vi "Phase unwrap (degrees).vi"(1 "Phase Shift (phy)\n(degrees)":dbl format="%#_6f") -> (0 "Degree":dbl)   [LabVIEW 2009]
panel:
  out "Principal value of\nphase shift":dbl
  out "(radians)":dbl
  # "radian"
  # "="
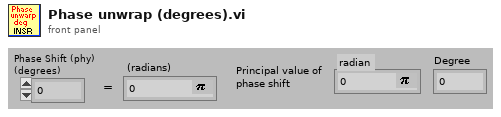
[diagram p1: front panel]
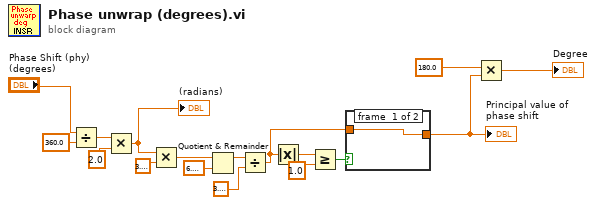
[diagram p0: block diagram]
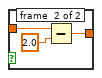
[diagram p2: hidden frame]
diagram:
  n1 = Divide(x="Phase Shift (phy)\n(degrees)", y=360.0 ("x")) -> (x/y=w16:dbl)
  n2 = Multiply(x=w16, y=2.0 ("x")) -> (x*y=w11:dbl)
  "(radians)" <- w11
  n3 = Multiply(x=w11, y=3.141592653589793) -> (x*y=w12:dbl)
  n4 = Quotient & Remainder(x=w12, y=6.283185307179586) -> (x-y*floor(x/y)=w13:dbl)  [unwired: 1 out]
  n5 = Divide(x=w13, y=3.141592653589793) -> (x/y=w5:dbl)
  n6 = Absolute Value(x=w5) -> (abs(x)=w4:dbl)
  n7 = Greater Or Equal?(x=w4, y=1.0 ("x")) -> (x >= y?=w6:bool)
  n8 = case shown="True" w6 {
    tunnel: w5 -> [w18 w21]
    tunnel: [w18 w20] -> w2
    frame #0 {
    }
    frame #1 {
      n9 = Subtract(x=w21, y=2.0 ("x")) -> (x-y=w20:dbl)
    }
  }
  "Principal value of\nphase shift" <- w2
  n10 = Multiply(x=180.0, y=w2) -> (x*y=→"Degree":dbl)
